vi "Export Data Items Nodes.vi"(8 "error in (no error)":errorcluster, 11 "Node Ptr":u64 format="%.0x") -> (0 "error out":errorcluster)   [LabVIEW 2023, in "Vires VTD System Explorer.lvlib"]
uses:
  Vires VTD System Explorer.lvlib
  <vilib>/Utility/xml.llb/Write to XML File(string).vi
  <vilib>/NI VeriStand/Custom Device Tools/Custom Device Utility Library/Custom Device Utility Library.lvlib
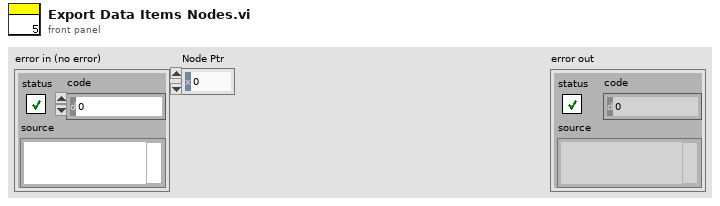
[diagram p1: front panel]
types:
  T1 = typedef "Vires VTD System Explorer.lvlib/Item Informations.ctl" = cluster{"Parents Section Names":string[], "Item Info":T2, "Channel Info":T3, "Data Channel Property":T5}
  T2 = typedef "Custom Device API.lvlib/Custom Device Item Info.ctl" = cluster{"Name":string, "Is Channel":bool, "GUID":string, "Is Waveform":bool}
  T3 = typedef "Custom Device API.lvlib/Custom Device Channel.ctl" = cluster{"Type":T4, "Units":string, "Default Value":dbl, "Faultable":bool, "Scalable":bool}
  T4 = typedef "Custom Device API.lvlib/Custom Device Channel Type.ctl" = enum16{"Input", "Output"}
  T5 = typedef "Vires VTD System Explorer.lvlib/Data Channel Custom Property.ctl" = cluster{"pkid":u32, "Signalname":string, "PlayerID":u8, "WheelID":i32}
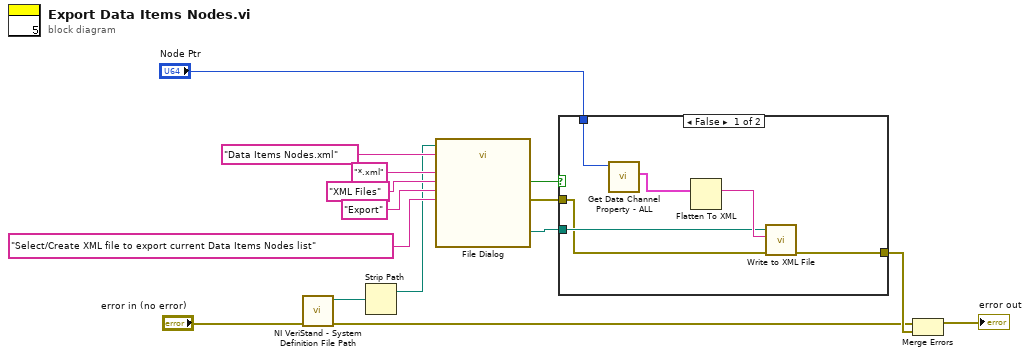
[diagram p0: block diagram]
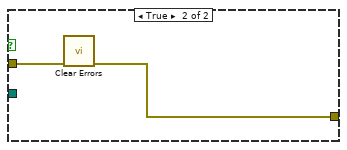
[diagram p2: hidden frame]
diagram:
  n1 = call <vilib>:"NI VeriStand - System Definition File Path.vi"("error in (no error)"="error in (no error)") -> ("error out"=w2:errorcluster, "SDF path"=w4:path)  [unwired: 9 in]
  n2 = Strip Path(path=w4) -> (stripped path=w1:path)  [unwired: 1 out]
  n3 = call "File Dialog"("start path"=w1, "prompt"="Select/Create XML file to export current Data Items Nodes list", "button label"="Export", "default name"="Data Items Nodes.xml", "pattern (all files)"="*.xml", "pattern label"="XML Files") -> ("selected path"=w9:path, "cancelled"=w10:bool, "error out"=w8:errorcluster)  [unwired: 6 in, 1 out]
  n4 = case shown="False" w10 {
    tunnel: w9 -> [w18 _]
    tunnel: w8 -> [w16 w23]
    tunnel: [w17 w22] -> w7
    tunnel: "Node Ptr" -> [w21 _]
    frame False {
      n5 = call "Get Data Channel Property - ALL.vi"("Item Ref in"=w21) -> ("Item Informations array(parsed)"=w20:T1[])  [unwired: 8 in, 2 out]
      n6 = Flatten To XML(6:w20) -> (2:w19:string)
      n7 = call-poly <vilib>:"Write to XML File.vi"("error in (no error)"=w16, "XML Input"=w19, "XML File Path"=w18) -> ("error out"=w17:errorcluster)  [unwired: 6 in, 2 out]
    }
    frame True {
      n8 = call <vilib>:"Clear Errors.vi"("error in (no error)"=w23) -> ("error out"=w22:errorcluster)  [unwired: 5 in, 1 out]
    }
  }
  n9 = Merge Errors(w2, w7) -> (→"error out":errorcluster)
